vi "CHROMA Initialize.vi"(5 "Phase Shift Lines":T1, 7 "Phase Shift Angle":i32=180, 8 "Error In":errorcluster, 9 "Voltage Limit":i32=130, 10 "Voltage Range":T2=enum."Low (150V)", 11 "CHROMA VISA In":refnum<visa-resource-name>) -> (0 "Error Out":errorcluster, 2 "Instrument Name":string, 3 "CHROMA VISA Out":refnum<visa-resource-name>)   [LabVIEW 2019]
uses:
  Type Definition/CHROMA Voltage Range.ctl
  Type Definition/CHROMA Phase Shift Lines.ctl
  <vilib>/Instr/_visa.llb/VISA Open Access Mode.ctl
  Type Definition/CHROMA Output State.ctl
  Type Definition/CHROMA Set Coupling.ctl
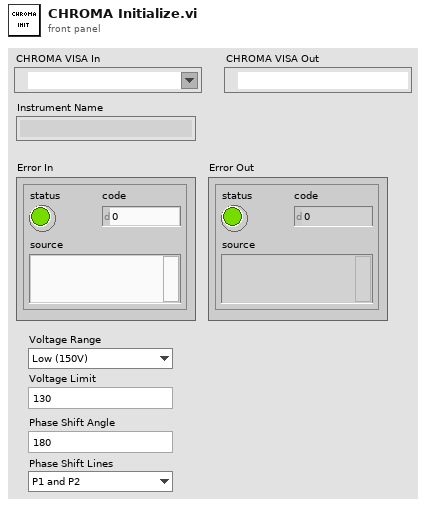
[diagram p1: front panel]
types:
  T1 = typedef "CHROMA Phase Shift Lines.ctl" = enum16{"P1 and P2", "P1 and P3"}
  T2 = typedef "CHROMA Voltage Range.ctl" = enum16{"High (300V)", "Low (150V)"}
  T3 = typedef "CHROMA Set Coupling.ctl" = enum16{"NONE", "ALL"}
  T4 = typedef "CHROMA Output State.ctl" = enum16{"Chroma OFF", "Chroma ON"}
  T5 = typedef "VISA Open Access Mode.ctl" = u32
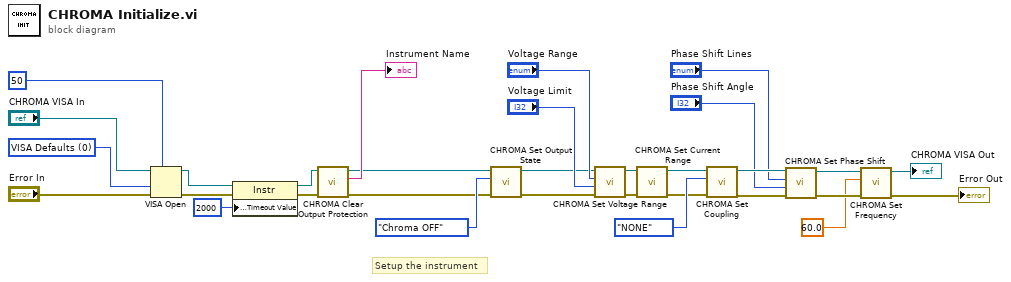
[diagram p0: block diagram]
diagram:
  w26 = T5 0 items=["VISA Defaults"=0, "Exclusive Lock"=1, "Load Configured Settings"=4] ("Access Mode")
  # "Setup the instrument"
  n1 = VISA Open(timeout (0)=u32 50 ("VISA Open timeout (0)"), access mode=w26, error in (no error)="Error In", VISA resource name="CHROMA VISA In") -> (VISA resource name=w24:refnum<visa-resource-name>, error out=w25:errorcluster)  [unwired: 1 in]
  n2 = property class="Instr"(reference=w24, error in=w25, "General Settings:Timeout Value"=u32 2000) -> (reference out=w6:refnum<visa-resource-name>, error out=w21:errorcluster)
  n3 = call "CHROMA Clear Output Protection.vi"("Error In"=w21, "CHROMA VISA In"=w6) -> ("Error Out"=w10:errorcluster, "Instrument Name"=→"Instrument Name":string, "CHROMA VISA Out"=w7:refnum<visa-resource-name>)  [unwired: 7 in]
  n4 = call "CHROMA Set Output State.vi"("Error In"=w10, "Chroma Output State"=CHROMA_Output_State."Chroma OFF", "CHROMA VISA In"=w7) -> ("Error Out"=w9:errorcluster, "CHROMA VISA Out"=w8:refnum<visa-resource-name>)  [unwired: 6 in, 1 out]
  n5 = call "CHROMA Set Voltage Range.vi"("Error In"=w9, "Voltage Limit"="Voltage Limit", "Voltage Range"="Voltage Range", "CHROMA VISA In"=w8) -> ("Error Out"=w30:errorcluster, "CHROMA VISA Out"=w31:refnum<visa-resource-name>)  [unwired: 6 in]
  n6 = call "CHROMA Set Current Range.vi"("Error In"=w30, "CHROMA VISA In"=w31) -> ("Error Out"=w11:errorcluster, "CHROMA VISA Out"=w12:refnum<visa-resource-name>)  [unwired: 8 in]
  n7 = call "CHROMA Set Coupling.vi"("Error In"=w11, "Chroma Couple"=CHROMA_Set_Coupling."NONE", "CHROMA VISA In"=w12) -> ("Error Out"=w17:errorcluster, "CHROMA VISA Out"=w18:refnum<visa-resource-name>)  [unwired: 7 in]
  n8 = call "CHROMA Set Phase Shift.vi"("Error In"=w17, "Value"="Phase Shift Angle", "Phase Shift Lines"="Phase Shift Lines", "CHROMA VISA In"=w18) -> ("Error Out"=w5:errorcluster, "CHROMA VISA Out"=w3:refnum<visa-resource-name>)  [unwired: 6 in]
  n9 = call "CHROMA Set Frequency.vi"("Error In"=w5, "Frequency"=60.0, "CHROMA VISA In"=w3) -> ("Error Out"=→"Error Out":errorcluster, "CHROMA VISA Out"=→"CHROMA VISA Out":refnum<visa-resource-name>)  [unwired: 7 in]
